vi "Query Status Register.vi"(8 "error in":errorcluster, 11 "6700C in":refnum<class "6700C.lvclass">) -> (0 "error out":errorcluster, 3 "6700C out":refnum<class "6700C.lvclass">)   [LabVIEW 2019, in "6700C.lvlib" / "6700C.lvclass"]
uses:
  Library/6700C.lvclass
  C:/Users/Public/Documents/Development/builds/Instruments/PowerSupply.lvlibp/Library/PowerSupply.lvclass
  builds/Instruments/PowerSupply.lvlibp/Private/Accessors/Read Number of Channels.vi
  builds/Instruments/PowerSupply.lvlibp/Accessors/Write Status Flags.vi
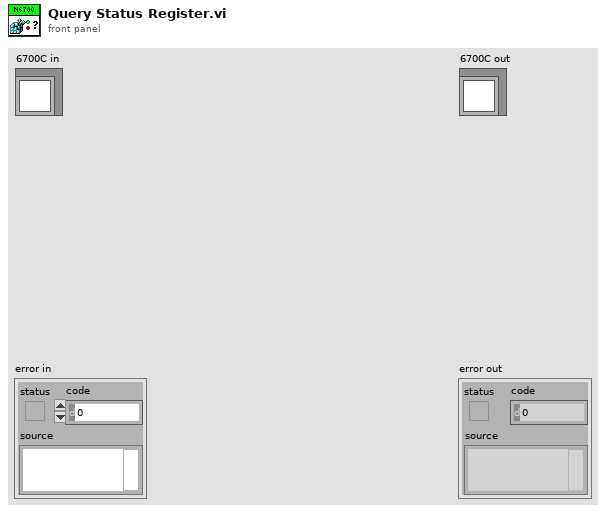
[diagram p1: front panel]
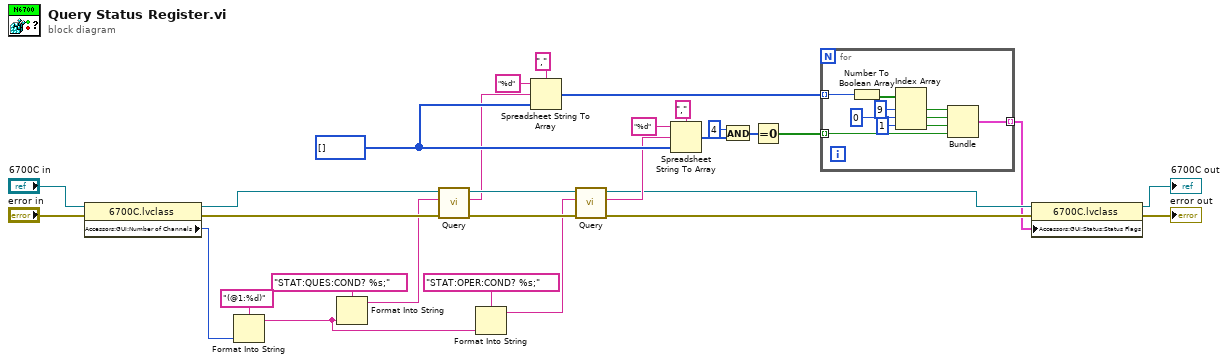
[diagram p0: block diagram]
diagram:
  w15 = u32[] []
  n1 = property class="6700C.lvclass"(reference="6700C in", error in="error in") -> (reference out=w25:refnum<class "6700C.lvclass">, error out=w27:errorcluster, "Accessors:GUI:Number of Channels"=w28:i32)
  n2 = Format Into String(format string="(@1:%d)", w28) -> (resulting string=w23:string)  [unwired: 2 in, 1 out]
  n3 = Format Into String(format string="STAT:QUES:COND? %s;", w23) -> (resulting string=w24:string)  [unwired: 2 in, 1 out]
  n4 = call "Query.vi"("error in"=w27, "Write in"=w24, "6700C in"=w25) -> ("error out"=w26:errorcluster, "Read out"=w6:string, "6700C out"=w21:refnum<class "6700C.lvclass">)  [unwired: 6 in]
  n5 = Format Into String(format string="STAT:OPER:COND? %s;", w23) -> (resulting string=w22:string)  [unwired: 2 in, 1 out]
  n6 = Spreadsheet String To Array(delimiter (Tab)=",", format string="%d", spreadsheet string=w6, array type (2D Dbl)=w15) -> (array=w11:u32[])
  n7 = call "Query.vi"("error in"=w26, "Write in"=w22, "6700C in"=w21) -> ("error out"=w5:errorcluster, "Read out"=w7:string, "6700C out"=w4:refnum<class "6700C.lvclass">)  [unwired: 6 in]
  n8 = Spreadsheet String To Array(delimiter (Tab)=",", format string="%d", spreadsheet string=w7, array type (2D Dbl)=w15) -> (array=w13:u32[])
  n9 = And(x=4, y=w13) -> (x .and. y?=w12:u32[])
  n10 = Equal To 0?(x=w12) -> (x = 0?=w10:bool[])
  n11 = for {
    tunnel: w11 -> [w40] mode=indexing
    tunnel: w10 -> [w35] mode=indexing
    tunnel: [w31] -> w3 mode=indexing
    n12 = Number To Boolean Array(number=w40) -> (Boolean array=w39:bool[])
    n13 = Index Array(array=w39, index #1=9 ("index"), index #2=0 ("index"), index #3=1 ("index")) -> (element #1=w32:bool, element #2=w33:bool, element #3=w34:bool)
    n14 = Bundle(w32, w33, w34, w35) -> (w31:cluster{bool, bool, bool, bool})  [unwired: 1 in]
  }
  n15 = property class="6700C.lvclass"(reference=w4, error in=w5, "Accessors:GUI:Status:Status Flags"=w3) -> (reference out=→"6700C out":refnum<class "6700C.lvclass">, error out=→"error out":errorcluster)
